vi "Initialise.vi"(8 "error in (no error)":errorcluster, 9 "Angle to Turn":dbl, 10 "Wheel Angle":dbl, 11 "Speed":dbl) -> (0 "error out":errorcluster, 3 "TurnInstruction.lvclass":refnum<class "TurnInstruction.lvclass">)   [LabVIEW 2015, in "TurnInstruction.lvclass"]
uses:
  TurnInstruction.lvclass
  TurnInstruction.lvclass/TurnInstruction.ctl
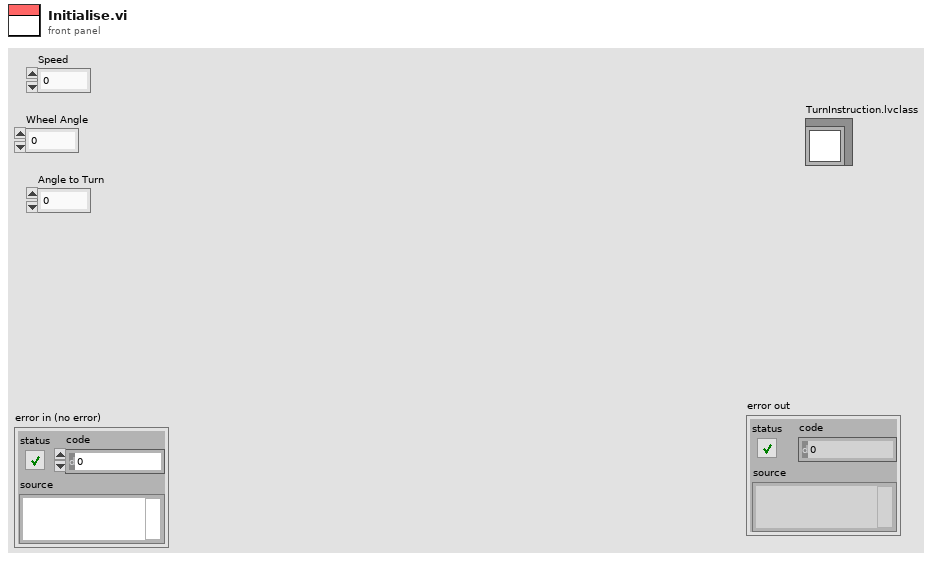
[diagram p1: front panel]
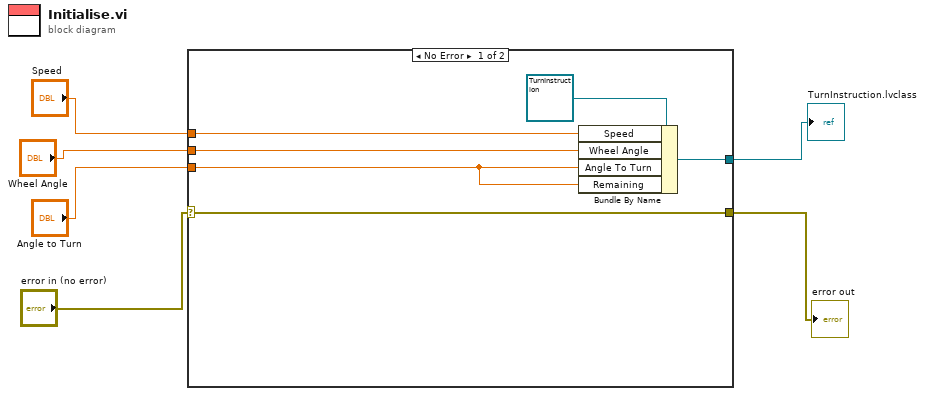
[diagram p0: block diagram]
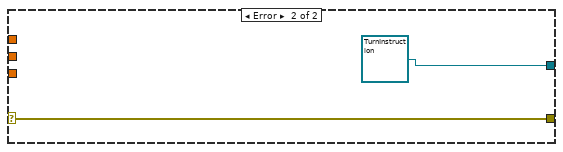
[diagram p2: hidden frame]
diagram:
  n1 = case shown="No Error" "error in (no error)" {
    selector: "error in (no error)" -> [w12 w14]
    tunnel: [w12 w14] -> w5
    tunnel: "Speed" -> [w10 _]
    tunnel: "Wheel Angle" -> [w9 _]
    tunnel: "Angle to Turn" -> [w8 _]
    tunnel: [w7 refnum<class "TurnInstruction.lvclass"> refnum ("TurnInstruction.lvclass")] -> w1
    frame No Error {
      n2 = Bundle By Name(cluster=refnum<class "TurnInstruction.lvclass"> refnum ("TurnInstruction.lvclass"), "Speed"=w10, "Wheel Angle"=w9, "Angle To Turn"=w8, "Remaining"=w8) -> (w7:refnum<class "TurnInstruction.lvclass">)
    }
    frame Error {
    }
  }
  "TurnInstruction.lvclass" <- w1
  "error out" <- w5
